vi "executeCommand.vi"(8 "error in (no error)":errorcluster, 10 "command":string, 11 "Electrometer in":refnum<class "Electrometer.lvclass">) -> (0 "error out":errorcluster, 3 "Electrometer out":refnum<class "Electrometer.lvclass">)   [LabVIEW 2016, in "Electrometer.lvclass"]
uses:
  Electrometer.lvclass
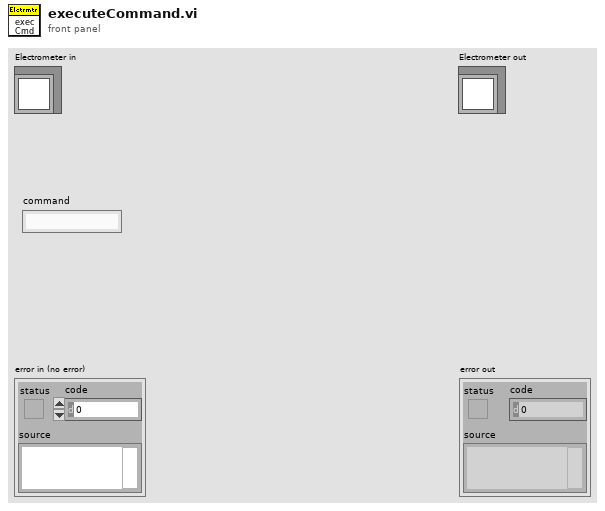
[diagram p1: front panel]
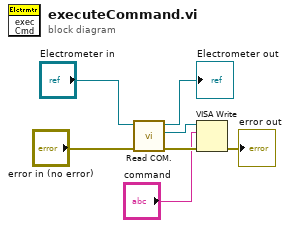
[diagram p0: block diagram]
diagram:
  n1 = call "Read COM..vi"("error in (no error)"="error in (no error)", "Electrometer in"="Electrometer in") -> ("error out"=w7:errorcluster, "VISA"=w6:refnum<visa-resource-name>, "Electrometer out"=→"Electrometer out":refnum<class "Electrometer.lvclass">)  [unwired: 7 in]
  n2 = VISA Write(VISA resource name=w6, write buffer="command", error in (no error)=w7) -> (error out=→"error out":errorcluster)  [unwired: 2 out]
